vi "Write configuration.vi"(8 "error in":errorcluster, 10 "configuration":refnum<class "NISE_CEF_serializable configuration.lvclass">, 11 "CVT Engine Editor in":refnum<class "CVT Engine Editor.lvclass">) -> (0 "error out":errorcluster, 3 "CVT Engine Editor out":refnum<class "CVT Engine Editor.lvclass">)   [LabVIEW 2013, in "CVT Engine Editor.lvclass"]
uses:
  CVT Engine Editor.lvclass
  <vilib>/NI/Configuration Framework/serializable configuration/NISE_CEF_serializable configuration.lvclass
  Configuration/CVT Engine Configuration.lvclass
  CVT Engine Editor.lvclass/CVT Engine Editor.ctl
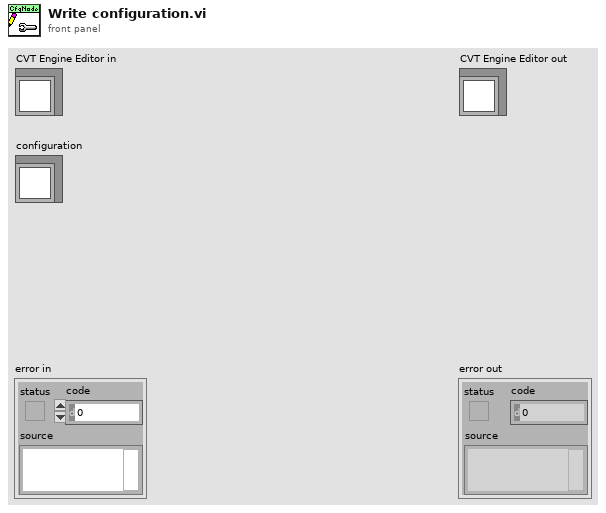
[diagram p1: front panel]
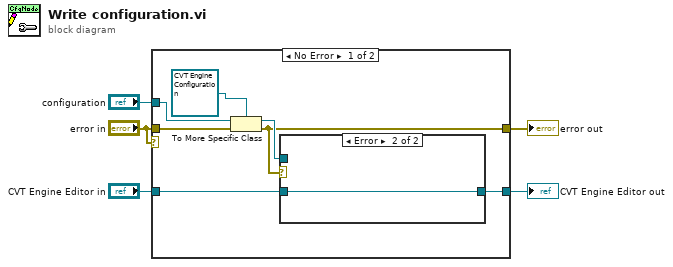
[diagram p0: block diagram]
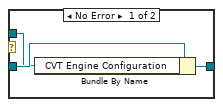
[diagram p2: hidden frame]
diagram:
  n1 = case shown="No Error" "error in" {
    tunnel: "error in" -> [w12 w18]
    tunnel: "CVT Engine Editor in" -> [w11 w17]
    tunnel: [w10 w17] -> w4
    tunnel: "configuration" -> [w9 _]
    tunnel: [w6 w18] -> w2
    frame No Error {
      n2 = To More Specific Class(target class=refnum<class "CVT Engine Configuration.lvclass"> refnum ("CVT Engine Configuration"), reference=w9, error in=w12) -> (specific class reference=w8:refnum<class "CVT Engine Configuration.lvclass">, error out=w6:errorcluster)
      n3 = case shown="Error" w6 {
        tunnel: w11 -> [w15 w16]
        tunnel: [w14 w16] -> w10
        tunnel: w8 -> [w13 _]
        frame No Error {
          n4 = Bundle By Name(cluster=w15, "CVT Engine Configuration"=w13) -> (w14:refnum<class "CVT Engine Editor.lvclass">)
        }
        frame Error {
        }
      }
    }
    frame Error {
    }
  }
  "error out" <- w2
  "CVT Engine Editor out" <- w4
